vi "VisaRead.vi"(2 "command":string=":FUNC:ON?", 3 "VISA资源名称":refnum<visa-resource-name>="GPIB0::24::INSTR") -> (0 "data":dbl format="%#_10g", 1 "read":string)   [LabVIEW 2014]
panel:
  out "错误输出":errorcluster
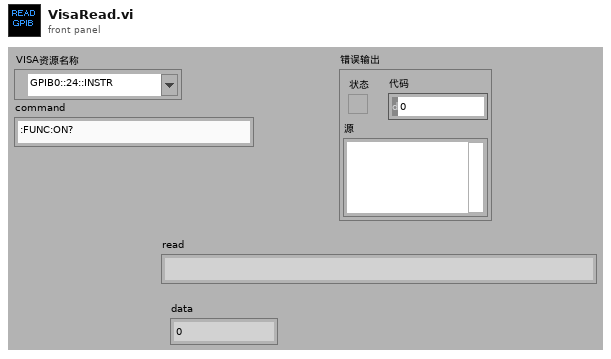
[diagram p1: front panel]
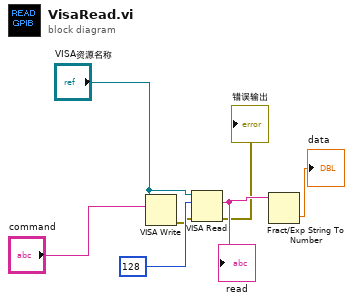
[diagram p0: block diagram]
diagram:
  n1 = VISA Write(VISA resource name="VISA资源名称", write buffer="command") -> (error out=w4:errorcluster)  [unwired: 1 in, 2 out]
  n2 = VISA Read ("VISA读取")(VISA resource name="VISA资源名称", byte count=u32 128 ("字节总数"), error in (no error)=w4) -> (read buffer=w6:string, error out=→"错误输出":errorcluster)  [unwired: 2 out]
  "read" <- w6
  n3 = Fract/Exp String To Number(string=w6) -> (number=→"data":dbl)  [unwired: 3 in, 1 out]
